vi "test_Create MetaData Channel_single channel type cast.vi"(8 "error in (no error)":errorcluster, 11 "TestCase in":refnum<class "Instrument Addon Scripting API Channels Unit Tests.lvclass">) -> (0 "error out":errorcluster, 3 "TestCase out":refnum<class "Instrument Addon Scripting API Channels Unit Tests.lvclass">)   [LabVIEW 2018, in "Instrument Addon Scripting API Channels Unit Tests.lvclass"]
uses:
  Instrument Addon Scripting API Channels Unit Tests.lvclass
  Addon/Addon Shared/Types/FG Control.ctl
  APIs/Scripting API/TypeDefs/Single Channel Type Cast Settings.ctl
  Addon/Addon Shared/Types/Type Cast Type.ctl
  Addon/Addon Shared/Types/Endian.ctl
  Instrument Addon Scripting API Channels Unit Tests.lvclass/Instrument Addon Scripting API Channels Unit Tests.ctl
  Addon/Addon Shared/SubVIs/Constants.vi
  <vilib>/NI Veristand/Custom Device Tools/Custom Device Utility Library/NI VeriStand - Search for Item by Name.vi
  APIs/Scripting API/Channels/Create MetaData Channel - Single Channel - Type Cast.vi
  <vilib>/NI Veristand/Custom Device Tools/Custom Device Utility Library/NI VeriStand - Search for Item by GUID.vi
  <vilib>/NI Veristand/Custom Device API/NI VeriStand - Get Item Property.vi
  <vilib>/NI Veristand/Custom Device API/Get Item Property (U32).vi
  <vilib>/NI Veristand/Custom Device API/Get Item Property (String Array).vi
  <vilib>/NI Veristand/Custom Device API/Get Item Property (String).vi
  <vilib>/NI Veristand/Custom Device API/NI VeriStand - Set Item Property.vi
  <vilib>/NI Veristand/Custom Device API/Set Item Property (U32).vi
  <vilib>/NI Veristand/Custom Device API/Set Item Property (String Array).vi
  <vilib>/NI Veristand/Custom Device API/NI VeriStand - Get Item Children.vi
  Addon/Addon Shared/SubVIs/Set Channel Value Table.vi
  <vilib>/NI Veristand/Custom Device API/Set Item Property (String).vi
  <vilib>/addons/_JKI Toolkits/VI Tester/TestCase.llb/TestCase.lvclass
  Instrument Addon Scripting API Test Assets/Instrument Addon Scripting API Test Assets.lvclass
  <vilib>/NI Veristand/Custom Device Tools/Custom Device Utility Library/Custom Device Utility Library.lvlib
  Addon/Addon Shared/Instrument Addon Shared.lvlib
  <vilib>/NI Veristand/Custom Device API/Custom Device API.lvlib
  APIs/Scripting API/Instrument Addon Scripting API.lvlib
  C:/Program Files (x86)/National Instruments/LabVIEW 2018/vi.lib/addons/_JKI Toolkits/VI Tester/TestCase.llb/TestCase.lvclass
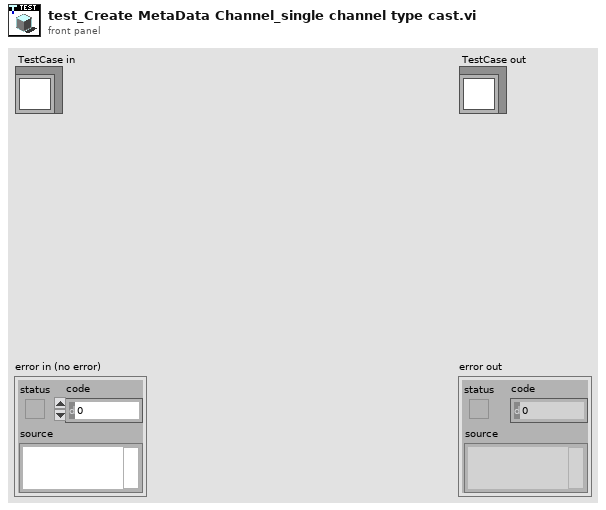
[diagram p1: front panel]
types:
  T1 = typedef "Instrument Addon Shared.lvlib/FG Control.ctl" = enum16{"Get", "Set"}
  T2 = typedef "Instrument Addon Scripting API.lvlib/Single Channel Type Cast Settings.ctl" = cluster{"Type":T3, "Endian":T4, "Default Value":dbl, "Units":string}
  T3 = typedef "Instrument Addon Shared.lvlib/Type Cast Type.ctl" = enum16{"DBL", "SGL", "U64", "U32", "U16", "U8", "I64", "I32", "I16", "I8"}
  T4 = typedef "Instrument Addon Shared.lvlib/Endian.ctl" = enum16{"Native", "Little", "Big"}
  T5 = typedef "Custom Device API.lvlib/Custom Device Item Ref.ctl" = u64
  T6 = typedef "Instrument Addon Shared.lvlib/MetaData Parameters.ctl" = cluster{"Data Type":T7, "Channel Type":T8, "List":string[], "Format String":string, "Type":T3, "Delimiter":string, "Endian":T4}
  T7 = typedef "Instrument Addon Shared.lvlib/Protocol Data Type.ctl" = enum16{"Single Channel", "Array"}
  T8 = typedef "Instrument Addon Shared.lvlib/Metadata Channel Type.ctl" = enum16{"Enumerated List", "Format", "Type Cast"}
  T9 = typedef "Custom Device API.lvlib/Custom Device Channel.ctl" = cluster{"Type":T10, "Units":string, "Default Value":dbl, "Faultable":bool, "Scalable":bool}
  T10 = typedef "Custom Device API.lvlib/Custom Device Channel Type.ctl" = enum16{"Input", "Output"}
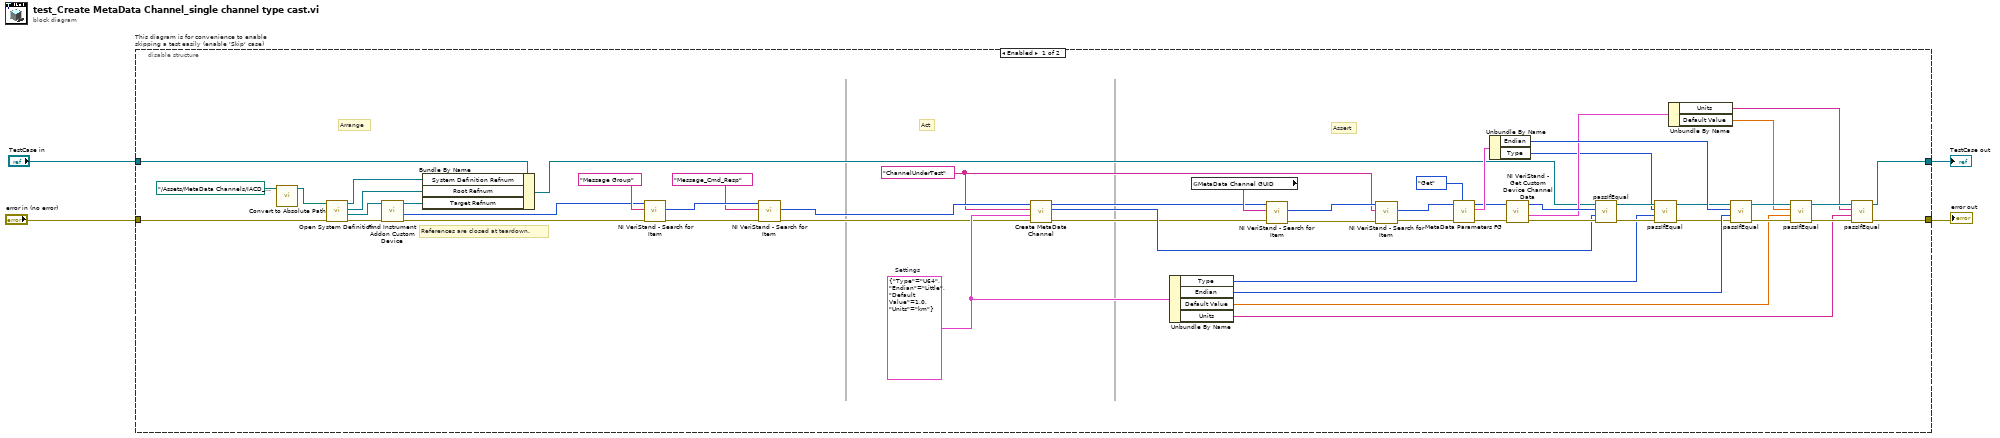
[diagram p0: block diagram]
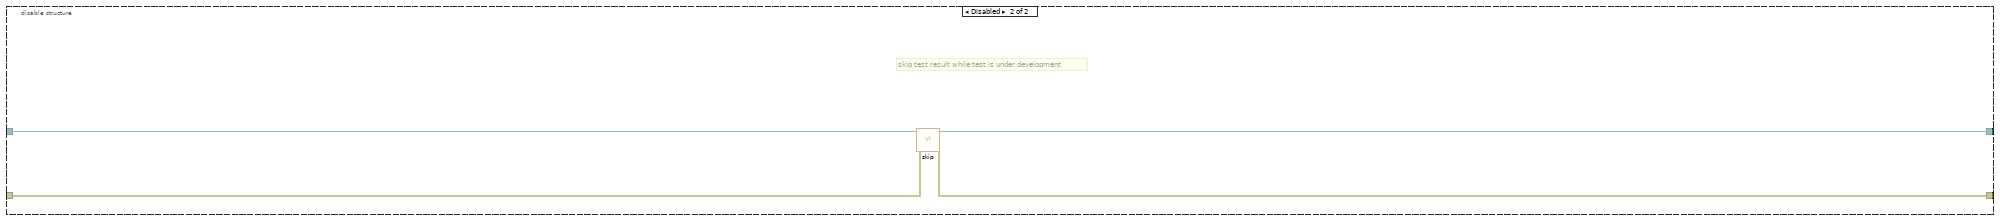
[diagram p2: hidden frame]
diagram:
  n1 = disable-structure "This diagram is for convenience to enable skipping a test easily (enable 'Skip' case)" shown="Enabled" {
    disable-tunnel: "TestCase in" -> [w26 w61]
    disable-tunnel: [w33 w59] -> w1
    disable-tunnel: [w32 w60] -> w3
    disable-tunnel: "error in (no error)" -> [w57 w58]
    frame Enabled {
      w11 = T2 {"Type"=enum."U64", "Endian"=enum."Little", "Default Value"=1.0, "Units"="km"}  # Settings
      w12 = "ChannelUnderTest" ("Name")
      # "References are closed at teardown."
      # "Assert"
      # "Act"
      # "Arrange"
      n2 = call "Convert to Absolute Path.vi"("System Definition File"=path "../Assets/MetaData Channels/IACD_channels.nivssdf") -> ("Absolute Path"=w5:path)  [unwired: 10 in]
      n3 = call "Open System Definition.vi"("error in (no error)"=w57, "System Definition File"=w5) -> ("error out"=w55:errorcluster, "Target Refnum"=w56:refnum<k24>, "Root Refnum"=w29:refnum<k24>, "System Definition Refnum"=w28:refnum<k24>)  [unwired: 6 in]
      n4 = call "Find Instrument Addon Custom Device.vi"("error in"=w55, "target in"=w56) -> ("error out"=w15:errorcluster, "NodeID"=w14:u64, "target out"=w30:refnum<k24>)  [unwired: 7 in]
      n5 = Bundle By Name(cluster=w26, "System Definition Refnum"=w28, "Root Refnum"=w29, "Target Refnum"=w30) -> (w27:refnum<class "Instrument Addon Scripting API Channels Unit Tests.lvclass">)
      n6 = call-poly <vilib>:"NI VeriStand - Search for Item.vi"("error in"=w15, "Item Name"="Message Group", "Section Ref in"=w14) -> ("error out"=w16:errorcluster, "Item Ref"=w18:T5)  [unwired: 5 in, 2 out]
      n7 = call-poly <vilib>:"NI VeriStand - Search for Item.vi"("error in"=w16, "Item Name"="Message_Cmd_Resp", "Section Ref in"=w18) -> ("error out"=w10:errorcluster, "Item Ref"=w13:T5)  [unwired: 5 in, 2 out]
      n8 = call-poly "Create MetaData Channel.vi"("Error In"=w10, "Settings"=w11, "Name"=w12, "Message Refnum In"=w13) -> ("Error Out"=w7:errorcluster, "Channel Refnum"=w8:T5, "Message Refnum Out"=w9:T5)  [unwired: 5 in]
      n9 = Unbundle By Name(w11) -> ("Type"=w21:T3, "Endian"=w42:T4, "Default Value"=w38:dbl, "Units"=w37:string)
      n10 = global read "Constants.vi" "MetaData Channel GUID"() -> (w54:string)
      n11 = call-poly <vilib>:"NI VeriStand - Search for Item.vi"("error in"=w7, "Item GUID"=w54, "Section Ref in"=w9) -> ("error out"=w52:errorcluster, "Item Ref"=w53:T5)  [unwired: 5 in, 2 out]
      n12 = call-poly <vilib>:"NI VeriStand - Search for Item.vi"("error in"=w52, "Item Name"=w12, "Section Ref in"=w53) -> ("error out"=w51:errorcluster, "Item Ref"=w50:T5)  [unwired: 5 in, 2 out]
      n13 = call "MetaData Parameters FG.vi"("Action"=FG_Control."Get", "error in (no error)"=w51, "Item Ref in"=w50) -> ("error out"=w40:errorcluster, "MetaData Parameters"=w48:T6, "Item Ref out"=w41:T5)  [unwired: 6 in]
      n14 = Unbundle By Name(w48) -> ("Endian"=w43:T4, "Type"=w20:T3)
      n15 = call <vilib>:"NI VeriStand - Get Custom Device Channel Data.vi"("error in (no error)"=w40, "Channel Ref in"=w41) -> ("error out"=w31:errorcluster, "Channel"=w36:T9, "Channel Ref out"=w39:T5)  [unwired: 4 in, 3 out]
      n16 = call-dynamic "passIfEqual.vi"("error in (no error)"=w31, "y"=w8, "x"=w39, "TestCase in"=w27) -> ("error out"=w25:errorcluster, "TestCase out"=w23:refnum<class "Instrument Addon Scripting API Channels Unit Tests.lvclass">)  [unwired: 6 in]
      n17 = call-dynamic "passIfEqual.vi"("error in (no error)"=w25, "y"=w21, "x"=w20, "TestCase in"=w23) -> ("error out"=w24:errorcluster, "TestCase out"=w22:refnum<class "Instrument Addon Scripting API Channels Unit Tests.lvclass">)  [unwired: 6 in]
      n18 = Unbundle By Name(w36) -> ("Units"=w34:string, "Default Value"=w35:dbl)
      n19 = call-dynamic "passIfEqual.vi"("error in (no error)"=w24, "y"=w42, "x"=w43, "TestCase in"=w22) -> ("error out"=w47:errorcluster, "TestCase out"=w46:refnum<class "Instrument Addon Scripting API Channels Unit Tests.lvclass">)  [unwired: 6 in]
      n20 = call-dynamic "passIfEqual.vi"("error in (no error)"=w47, "y"=w38, "x"=w35, "TestCase in"=w46) -> ("error out"=w45:errorcluster, "TestCase out"=w44:refnum<class "Instrument Addon Scripting API Channels Unit Tests.lvclass">)  [unwired: 6 in]
      n21 = call-dynamic "passIfEqual.vi"("error in (no error)"=w45, "y"=w37, "x"=w34, "TestCase in"=w44) -> ("error out"=w32:errorcluster, "TestCase out"=w33:refnum<class "Instrument Addon Scripting API Channels Unit Tests.lvclass">)  [unwired: 6 in]
    }
    frame Disabled {
      # "skip test result while test is under development"
      n22 = call <vilib>:"skip.vi"("error in (no error)"=w58, "TestCase in"=w61) -> ("error out"=w60:errorcluster, "TestCase out"=w59:refnum<class "Instrument Addon Scripting API Channels Unit Tests.lvclass">)  [unwired: 8 in]
    }
  }
  "error out" <- w3
  "TestCase out" <- w1
